vi "Réponse Opérateur Pédale.vi"(8 "errin":errorcluster, 10 "VISAin":refnum<visa-resource-name>, 11 "ex":string) -> (0 "errout":errorcluster, 1 "toute l'expression":string, 3 "ArrsurErr":bool)   [LabVIEW 2020]
doc: "Vérifie le retour d'une saisie en fonction d'une expression régulière"
uses:
  <vilib>/regexp/Match Regular Expression.xnode
panel:
  out "errout 2":errorcluster caption="errout"
  out "out":string
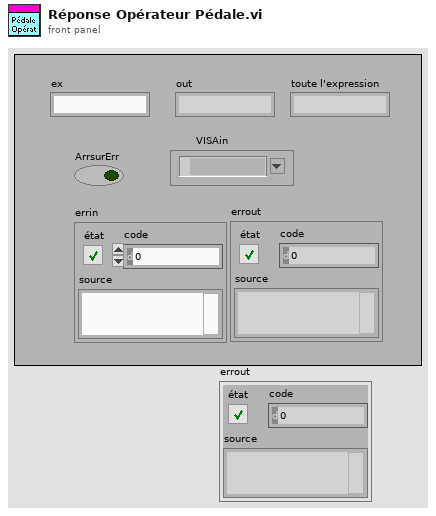
[diagram p1: front panel]
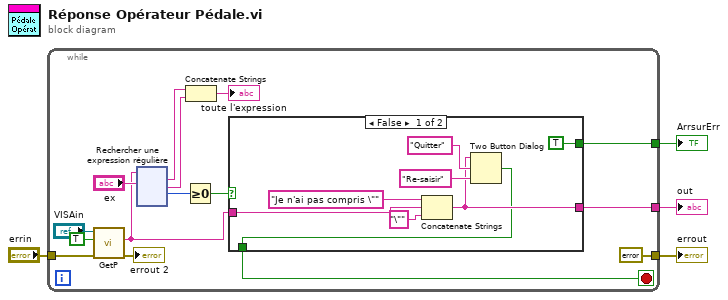
[diagram p0: block diagram]
diagram:
  n1 = while {
    tunnel: "errin" -> [w11]
    tunnel: [w19] -> w4
    tunnel: [errorcluster {"status"=FALSE, "code"=0, "source"=""} ("errout")] -> w1
    tunnel: [w18] -> w3
    stop <- w8 stop-if-true
    n2 = call <userlib>:"GetP.vi"("errin"=w11, "Pédale ON?"=TRUE, "VISAin"="VISAin") -> ("errout"=→"errout 2":errorcluster, "Data out"=w10:string)  [unwired: 7 in]
    n3 = xnode "Rechercher une expression régulière"("chaîne en entrée"=w10, "expression régulière"="ex") -> ("toute l'expression"=w14:string, "après la correspondance"=w13:string, "offset après correspondance"=w15:i32)  [unwired: 4 in, 2 out]
    n4 = Greater Or Equal To 0?(x=w15) -> (x >= 0?=w17:bool)
    n5 = Concatenate Strings(w14, w13) -> (→"toute l'expression":string)
    n6 = case shown="False" w17 {
      selector: w17 -> [_ w142]
      tunnel: [TRUE _] -> w19
      tunnel: w10 -> [w136 w143]
      tunnel: [w135 w143] -> w18
      tunnel: [w134 w142] -> w8
      frame False {
        n7 = Concatenate Strings("Je n'ai pas compris \"" ("message"), w136, "\"" ("chaîne")) -> (w135:string)
        n8 = Two Button Dialog(message=w135, 1:"Re-saisir" ("Nom du bouton V (\"OK\")"), 2:"Quitter" ("Nom du bouton F (\"Annuler\")")) -> (T button?=w134:bool)
      }
      frame True {
      }
    }
  }
  "ArrsurErr" <- w4
  "errout" <- w1
  "out" <- w3
